vi "DSF.Engine.Pool.Plugin Interface.Obtain from Pool.vi"(2 "Plugin Interface":refnum<class "DSF.Engine.Interface.Plugin.lvclass">, 8 "error in (no error)":errorcluster, 11 "Plugin Interface Pool in":refnum<class "DSF.Engine.Pool.Plugin Interface.lvclass">) -> (0 "error out":errorcluster, 3 "Plugin Interface Pool out":refnum<class "DSF.Engine.Pool.Plugin Interface.lvclass">)   [LabVIEW 2016, in "DSF.Engine.lvlib" / "DSF.Engine.Pool.Plugin Interface.lvclass"]
uses:
  DSF.Engine.Pool.Plugin Interface.lvclass
  Interface/DSF.Engine.Interface.Plugin.lvclass
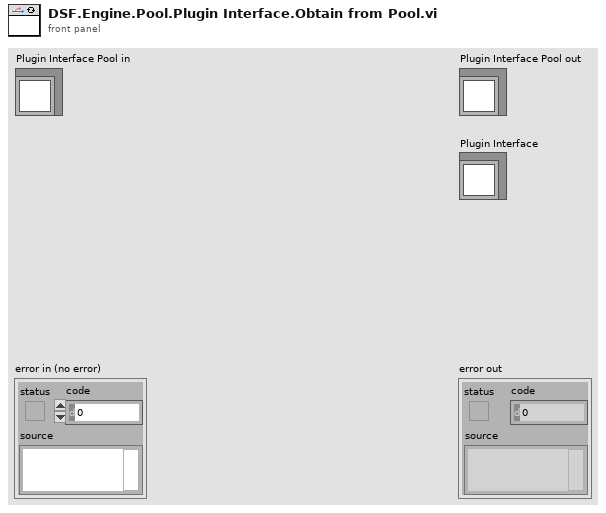
[diagram p1: front panel]
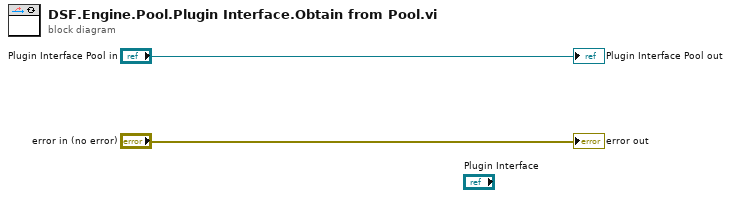
[diagram p0: block diagram]
diagram:
  "error out" <- "error in (no error)"
  "Plugin Interface Pool out" <- "Plugin Interface Pool in"
